vi "GetFreqRatio.vi"(8 "错误输入（无错误）":errorcluster, 11 "将要设置的分频比":u16) -> (0 "错误输出":errorcluster, 3 "返回值":u8)   [LabVIEW 2014]
uses:
  X86Dll/ZXUTConfigMgr.dll
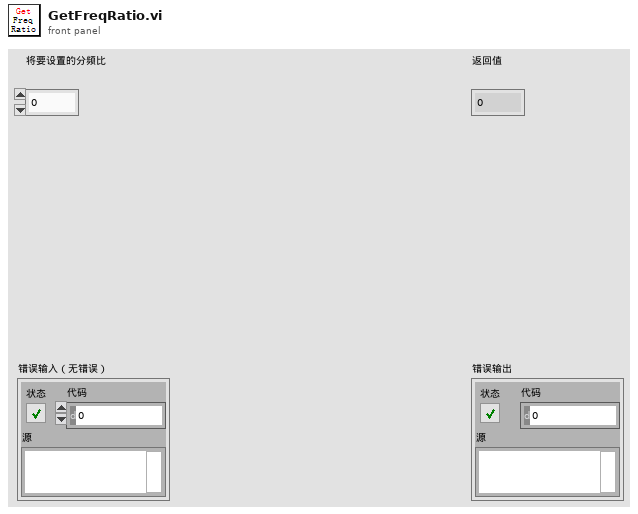
[diagram p1: front panel]
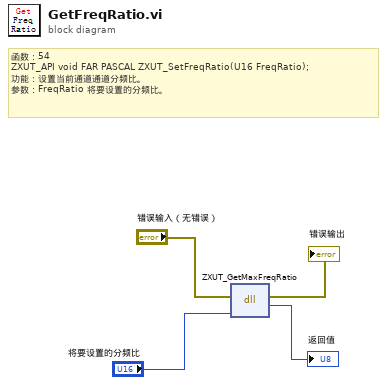
[diagram p0: block diagram]
diagram:
  # "函数：54\nZXUT_API void\tFAR PASCAL ZXUT_SetFreqRatio(U16 FreqRatio);\n功能：设置当前通道通道分频比。\n参数：FreqRatio 将要设置的分频比。"
  n1 = dll-call lib="D:/Software/Utrasonic on-line monitoring/X86Dll/ZXUTConfigMgr.dll" fn="ZXUT_GetMaxFreqRatio"(error in="错误输入（无错误）", "FreqRatio"="将要设置的分频比") -> (error out=→"错误输出":errorcluster, "返回值"=→"返回值":u8)  [unwired: 3 in, 1 out]
